vi "SetN2.vi"(8 "error in (no error)":errorcluster, 10 "Property":dbl, 11 "object in":refnum<class "Object (subject).lvclass">) -> (0 "error out":errorcluster, 3 "object out":refnum<class "Object (subject).lvclass">)   [LabVIEW 2014, in "Object (subject).lvclass"]
uses:
  Object (subject).lvclass
  Object (subject).lvclass/Object (subject).ctl
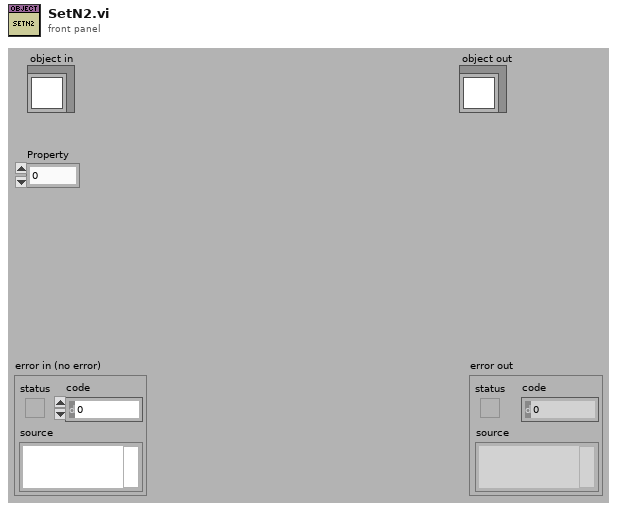
[diagram p1: front panel]
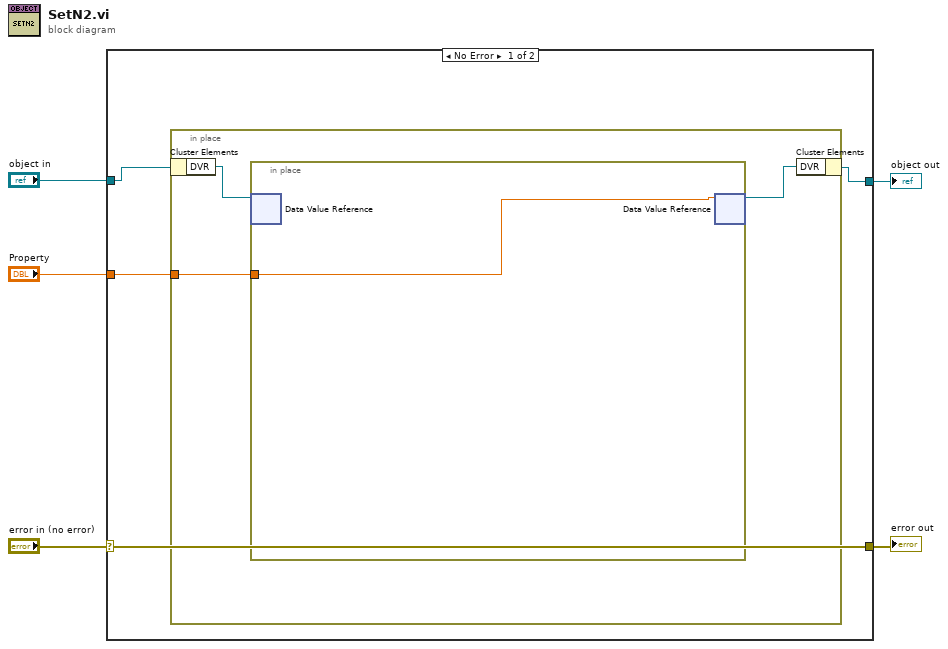
[diagram p0: block diagram]
diagram:
  n1 = case shown="No Error" "error in (no error)" {
    selector: "error in (no error)" -> [w9 w15]
    tunnel: [w9 w15] -> w4
    tunnel: [w7 w14] -> w2
    tunnel: "object in" -> [w8 w14]
    tunnel: "Property" -> [w6 _]
    frame No Error {
      n2 = in-place {
        in-place-border: w6 -> [w10]
        n3 = in-place-cluster #1(w8) -> ("DVR"=w12:refnum<data-value>)
        n4 = in-place {
          in-place-border: w10 -> [w13]
          n5 = in-place-dvr #2(w12) -> ()  [unwired: 2 out]
          n6 = in-place-dvr #2(w13) -> (w11:refnum<data-value>)  [unwired: 1 out]
        }
        n7 = in-place-cluster #1("DVR"=w11) -> (w7:refnum<class "Object (subject).lvclass">)
      }
    }
    frame Error {
    }
  }
  "error out" <- w4
  "object out" <- w2
